vi "Message Handler.vi"(11 "Consumer":refnum<class "Abstract Consumer.lvclass">) -> ()   [LabVIEW 2024, in "AIM ARINC 429 Engine.lvlib" / "Implementation.lvlib" / "Word Logging.lvlib"]
uses:
  Word Logging.lvlib
  <vilib>/NI/VeriStand Custom Device Messaging/Consumer/Abstract Consumer/Abstract Consumer.lvclass
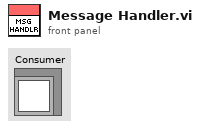
[diagram p1: front panel]
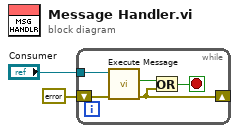
[diagram p0: block diagram]
diagram:
  n1 = while {
    tunnel: "Consumer" -> [w7]
    shift-right: [w3] -> _
    shift-left: errorcluster {"status"=FALSE, "code"=0, "source"=""} ("error in (no error)") -> [w4]
    stop <- w5 stop-if-true
    n2 = call <vilib>:"Execute Message.vi"("error in (no error)"=w4, "Abstract Consumer in"=w7) -> ("error out"=w3:errorcluster, "Stop?"=w6:bool)  [unwired: 6 in, 2 out]
    n3 = Or(x=w6, y=w3) -> (x .or. y?=w5:bool)
  }
